vi "Write TestConfiguration.vi"(8 "error in (no error)":errorcluster, 10 "TestLimit":string[][](array[string]), 11 "TestConfiguration in":refnum<class "TestConfiguration.lvclass">) -> (0 "error out":errorcluster, 3 "TestConfiguration out":refnum<class "TestConfiguration.lvclass">)   [LabVIEW 2019, in "TestSetup.lvlib" / "TestConfiguration.lvclass"]
uses:
  TestConfiguration.lvclass
  TestConfiguration.lvclass/TestConfiguration.ctl
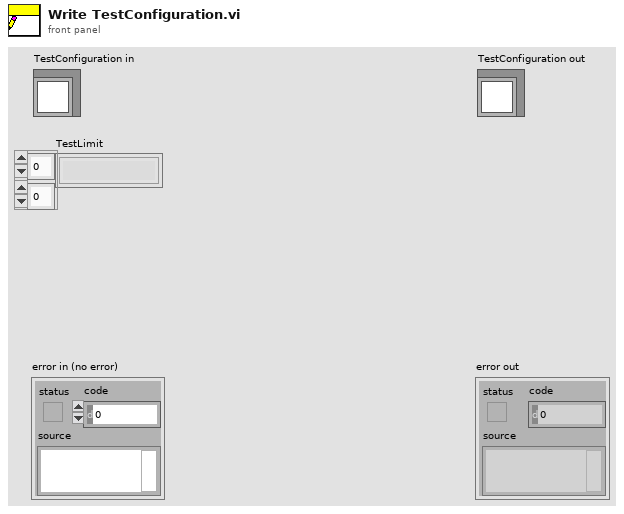
[diagram p1: front panel]
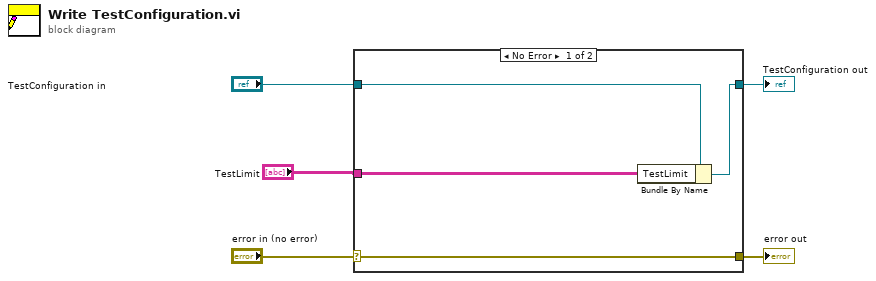
[diagram p0: block diagram]
diagram:
  n1 = case shown="No Error" "error in (no error)" {
    selector: "error in (no error)" -> [w9 w10]
    tunnel: [w9 w10] -> w4
    tunnel: [w7 w11] -> w2
    tunnel: "TestConfiguration in" -> [w8 w11]
    tunnel: "TestLimit" -> [w6 _]
    frame No Error {
      n2 = Bundle By Name(cluster=w8, "TestLimit"=w6) -> (w7:refnum<class "TestConfiguration.lvclass">)
    }
    frame Error {
    }
  }
  "error out" <- w4
  "TestConfiguration out" <- w2
